vi "BatteryMonitoringSystem.vi"() -> ()   [LabVIEW 2020]
uses:
  <vilib>/httpClient/LabVIEWHTTPClient.lvlib
panel:
  out "Battery temperature":dbl(slide) scale=0.0..100.0
  out "Temperature":dbl
  out "SOC":dbl
  out "Current":dbl
  out "Voltage":dbl
  in  "url":string
  # "Batter Monitoring System"
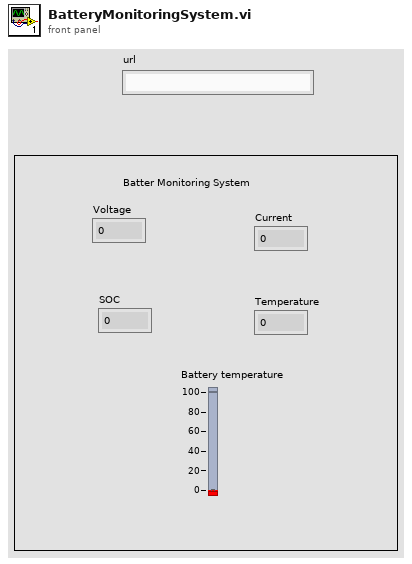
[diagram p1: front panel]
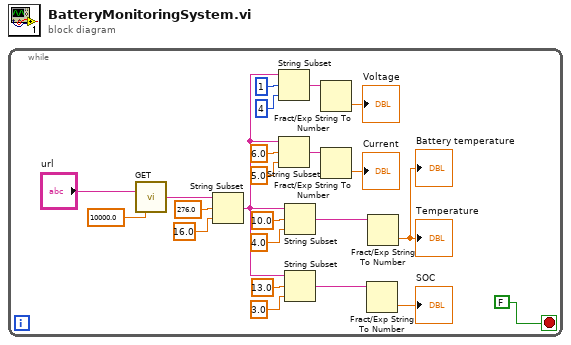
[diagram p0: block diagram]
diagram:
  n1 = while {
    stop <- FALSE stop-if-true
    n2 = call <vilib>:"GET.vi"("url"="url", "timeout (10000)"=10000.0 ("Numeric")) -> ("body"=w2:string)  [unwired: 10 in, 3 out]
    n3 = String Subset(string=w2, offset (0)=276.0 ("Numeric"), length (rest)=16.0 ("Numeric")) -> (substring=w1:string)
    n4 = String Subset(string=w1, offset (0)=1, length (rest)=4 ("length (rest)")) -> (substring=w12:string)
    n5 = String Subset(string=w1, offset (0)=6.0 ("Numeric"), length (rest)=5.0 ("Numeric")) -> (substring=w13:string)
    n6 = String Subset(string=w1, offset (0)=10.0 ("Numeric"), length (rest)=4.0 ("Numeric")) -> (substring=w8:string)
    n7 = String Subset(string=w1, offset (0)=13.0 ("Numeric"), length (rest)=3.0 ("Numeric")) -> (substring=w4:string)
    n8 = Fract/Exp String To Number(string=w12) -> (number=→"Voltage":dbl)  [unwired: 3 in, 1 out]
    n9 = Fract/Exp String To Number(string=w13) -> (number=→"Current":dbl)  [unwired: 3 in, 1 out]
    n10 = Fract/Exp String To Number(string=w4) -> (number=→"SOC":dbl)  [unwired: 3 in, 1 out]
    n11 = Fract/Exp String To Number(string=w8) -> (number=→"Temperature" →"Battery temperature":dbl)  [unwired: 3 in, 1 out]
  }
